vi "Scripting_FindControlsOnDiagram.vi"(0 "ViRef":refnum<vi>, 1 "TypeDefControlsToSerachFor":path[](array[path]), 2 "SearchAlsoBlockDiagram":bool, 5 "error in (no error)":errorcluster) -> (15 "FronPanelControlsFound":refnum<vi>[](array[refnum]), 16 "BlockDiagramConstantsFound":refnum<vi>[](array[refnum]), 19 "error out":errorcluster)   [LabVIEW 2014]
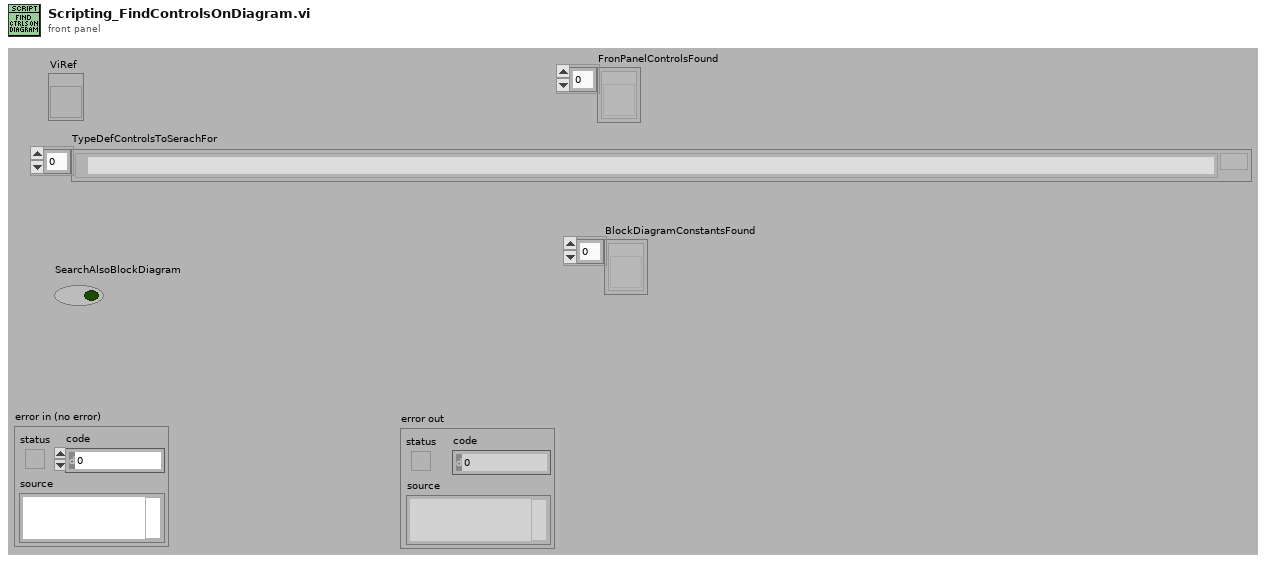
[diagram p1: front panel]
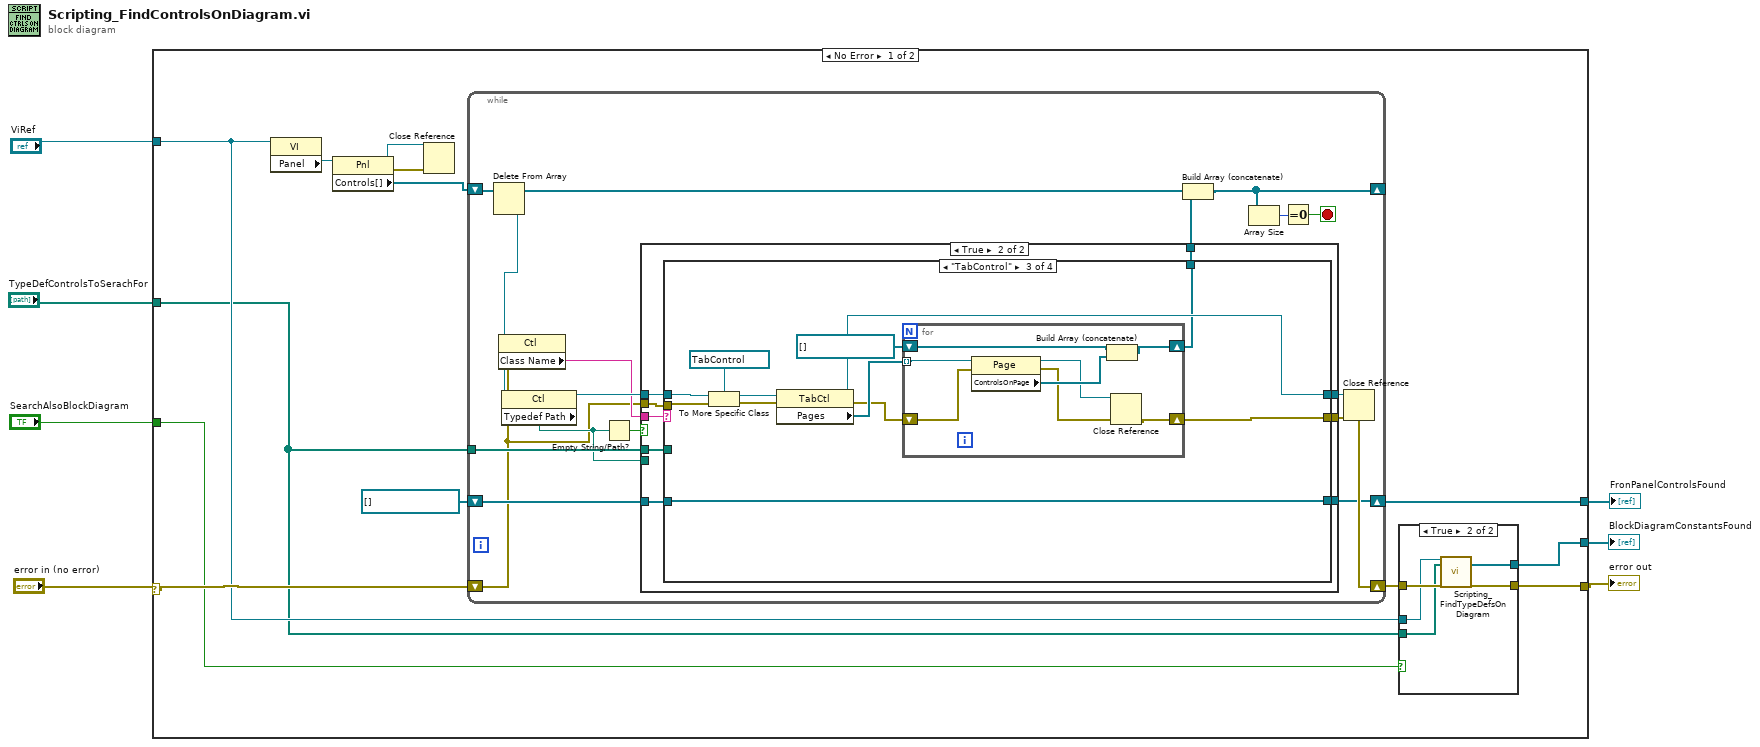
[diagram p0: block diagram]
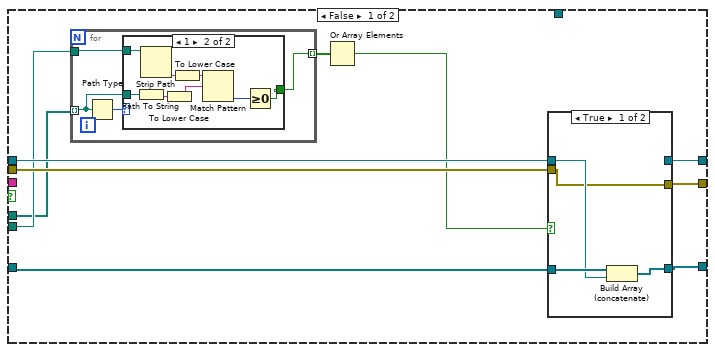
[diagram p3: hidden frame]
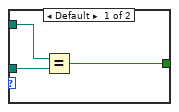
[diagram p4: hidden frame]
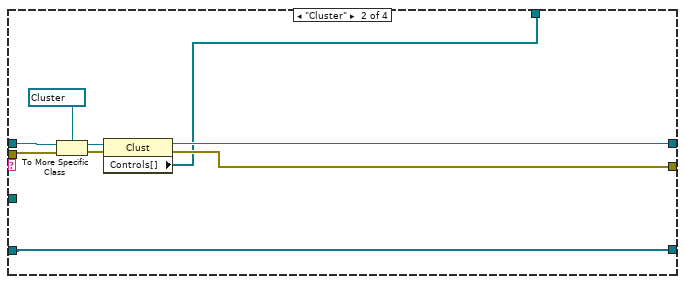
[diagram p7: hidden frame]
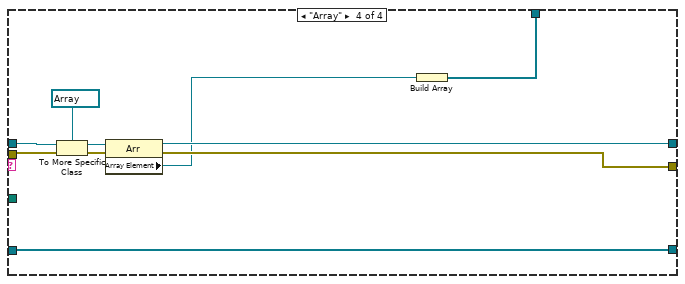
[diagram p8: hidden frame]
diagram:
  n1 = case shown="No Error" "error in (no error)" {
    selector: "error in (no error)" -> [w19 w127]
    tunnel: [w12 w127] -> w7
    tunnel: "TypeDefControlsToSerachFor" -> [w10 _]
    tunnel: "ViRef" -> [w11 _]
    tunnel: [w20 _] -> w3
    tunnel: "SearchAlsoBlockDiagram" -> [w9 _]
    tunnel: [w8 _] -> w1
    frame No Error {
      n2 = property class="VI"(reference=w11) -> ("Panel"=w16:refnum<vi>)  [unwired: 1 in, 2 out]
      n3 = property class="Pnl"(reference=w16) -> (reference out=w17:refnum<vi>, error out=w15:errorcluster, "Controls[]"=w18:refnum<vi>[])  [unwired: 1 in]
      n4 = Close Reference(reference=w17, error in (no error)=w15) -> ()  [unwired: 1 out]
      n5 = while {
        shift-right: [w38] -> _
        shift-left: w18 -> [w43]
        shift-right: [w35] -> w13
        shift-left: w19 -> [w27]
        tunnel: w10 -> [w36]
        shift-right: [w33] -> w20
        shift-left: refnum<vi>[] [] -> [w34]
        stop <- w41 stop-if-true
        n6 = Delete From Array(array=w43) -> (deleted portion=w29:refnum<vi>, array with subset deleted=w39:refnum<vi>[])  [unwired: 2 in]
        n7 = property class="Ctl"(reference=w29, error in=w27) -> ("Class Name"=w28:string)  [unwired: 2 out]
        n8 = property class="Ctl"(reference=w29, error in=w27) -> (reference out=w40:refnum<vi>, "Typedef Path"=w30:path)  [unwired: 1 out]
        n9 = Empty String/Path?(string/path=w30) -> (empty?=w32:bool)
        n10 = case shown="True" w32 {
          tunnel: w27 -> [w49 w84]
          tunnel: w40 -> [w51 w83]
          tunnel: [w48 w82] -> w37
          tunnel: w36 -> [w46 w81]
          tunnel: [w50 w80] -> w35
          tunnel: w34 -> [w53 w79]
          tunnel: [w52 w78] -> w33
          tunnel: w28 -> [_ w77]
          tunnel: [_ w76] -> w31
          tunnel: w30 -> [w47 _]
          frame False {
            n11 = for {
              tunnel: w46 -> [w56] mode=indexing
              tunnel: w47 -> [w55]
              tunnel: [w54] -> w44 mode=indexing
              n12 = Path Type(1:w56) -> (0:w57:i16)
              n13 = case shown="1" w57 {
                tunnel: w56 -> [w60 w68]
                tunnel: w55 -> [w59 w67]
                tunnel: [w58 w63] -> w54
                frame Default {
                  n14 = Equal?(x=w59, y=w60) -> (x = y?=w58:bool)
                }
                frame 1 {
                  n15 = Path To String(path=w68) -> (string=w65:string)
                  n16 = Strip Path(path=w67) -> (name=w66:string)  [unwired: 1 out]
                  n17 = To Lower Case(string=w65) -> (all lower case string=w61:string)
                  n18 = To Lower Case(string=w66) -> (all lower case string=w62:string)
                  n19 = Match Pattern(string=w62, regular expression=w61) -> (offset past match=w64:i32)  [unwired: 1 in, 3 out]
                  n20 = Greater Or Equal To 0?(x=w64) -> (x >= 0?=w63:bool)
                }
              }
            }
            n21 = Or Array Elements(Boolean array=w44) -> (logical OR=w45:bool)
            n22 = case shown="True" w45 {
              tunnel: w51 -> [w70 w75]
              tunnel: [_ w75] -> w48
              tunnel: [w69 w73] -> w50
              tunnel: w53 -> [w72 w74]
              tunnel: [w71 w74] -> w52
              tunnel: w49 -> [w69 w73]
              frame True {
                n23 = Build Array (concatenate)(w72, w70) -> (w71:refnum<vi>[])
              }
              frame False {
              }
            }
          }
          frame True {
            n24 = case shown="\"TabControl\"" w77 {
              tunnel: w83 -> [w86 w96 w108 w126]
              tunnel: w84 -> [w85 w92 w103 w122]
              tunnel: [w85 w89 w101 w120] -> w80
              tunnel: [_ w88 w99 w117] -> w76
              tunnel: [w86 w91 w102 w121] -> w82
              tunnel: w81 -> [_ _ _ _]
              tunnel: w79 -> [w87 w90 w98 w119]
              tunnel: [w87 w90 w98 w119] -> w78
              frame Default {
              }
              frame "Cluster" {
                n25 = To More Specific Class(target class=refnum<vi> refnum ("CaseSelector"), reference=w96, error in=w92) -> (specific class reference=w94:refnum<vi>, error out=w93:errorcluster)
                n26 = property class="Clust"(reference=w94, error in=w93) -> (reference out=w91:refnum<vi>, error out=w89:errorcluster, "Controls[]"=w88:refnum<vi>[])
              }
              frame "TabControl" {
                n27 = To More Specific Class(target class=refnum<vi> refnum ("CaseSelector"), reference=w108, error in=w103) -> (specific class reference=w106:refnum<vi>, error out=w104:errorcluster)
                n28 = property class="TabCtl"(reference=w106, error in=w104) -> (reference out=w102:refnum<vi>, error out=w100:errorcluster, "Pages"=w105:refnum<vi>[])
                n29 = for {
                  tunnel: w105 -> [w116] mode=indexing
                  shift-right: [w109] -> w101
                  shift-left: w100 -> [w115]
                  shift-right: [w112] -> w99
                  shift-left: refnum<vi>[] [] -> [w114]
                  n30 = property class="Page"(reference=w116, error in=w115) -> (reference out=w110:refnum<vi>, error out=w111:errorcluster, "ControlsOnPage"=w113:refnum<vi>[])
                  n31 = Build Array (concatenate)(w114, w113) -> (w112:refnum<vi>[])
                  n32 = Close Reference(reference=w110, error in (no error)=w111) -> (error out=w109:errorcluster)
                }
              }
              frame "Array" {
                n33 = To More Specific Class(target class=refnum<vi> refnum ("WhileLoop"), reference=w126, error in=w122) -> (specific class reference=w125:refnum<vi>, error out=w123:errorcluster)
                n34 = property class="Arr"(reference=w125, error in=w123) -> (reference out=w121:refnum<vi>, error out=w120:errorcluster, "Array Element"=w118:refnum<vi>)
                n35 = Build Array(w118) -> (w117:refnum<vi>[])
              }
            }
          }
        }
        n36 = Build Array (concatenate)(w39, w31) -> (w38:refnum<vi>[])
        n37 = Array Size(array=w38) -> (size(s)=w42:i32)
        n38 = Equal To 0?(x=w42) -> (x = 0?=w41:bool)
        n39 = Close Reference(reference=w37, error in (no error)=w35) -> ()  [unwired: 1 out]
      }
      n40 = case shown="True" w9 {
        tunnel: w13 -> [w21 w26]
        tunnel: [w21 w25] -> w12
        tunnel: w11 -> [_ w24]
        tunnel: w10 -> [_ w23]
        tunnel: [_ w22] -> w8
        frame False {
        }
        frame True {
          n41 = call <resource>:"Scripting_FindTypeDefsOnDiagram.vi"("ViRef"=w24, "TypeDefConstantsToSearchSearchFor"=w23, "error in (no error)"=w26) -> ("BlockDiagramConstantsFound"=w22:refnum<vi>[], "error out"=w25:errorcluster)  [unwired: 15 in]
        }
      }
    }
    frame Error {
    }
  }
  "error out" <- w7
  "FronPanelControlsFound" <- w3
  "BlockDiagramConstantsFound" <- w1
